vi "ULS ROI.vi"(8 "error in (no error)":errorcluster, 10 "ROI":cluster{"X1":sgl, "X2":sgl, "Y1":sgl, "Y2":sgl}, 11 "IFD in":refnum<class "IFD.lvclass">) -> (0 "error out":errorcluster, 3 "IFD out":refnum<class "IFD.lvclass">)   [LabVIEW 2016, in "IFD.lvclass"]
uses:
  IFD.lvclass
  Tag/IFD_Tag.lvclass/IFD_Tag.ctl
  IFD.lvclass/IFD.ctl
  Tag/IFD_Tag.lvclass
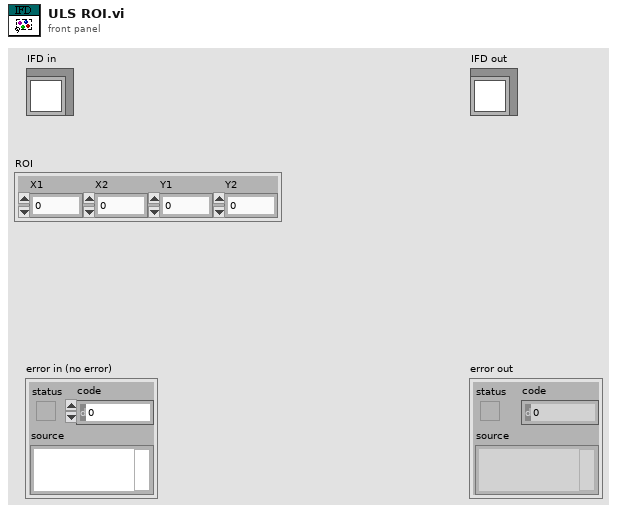
[diagram p1: front panel]
types:
  T1 = enum16{"Undefined(DO NOT USE)", "U8", "ASCII", "U16", "U32", "RATIONAL", "I8", "Undefined 8 bit", "I16", "I32", "SRATIONAL", "SGL", "DBL"}
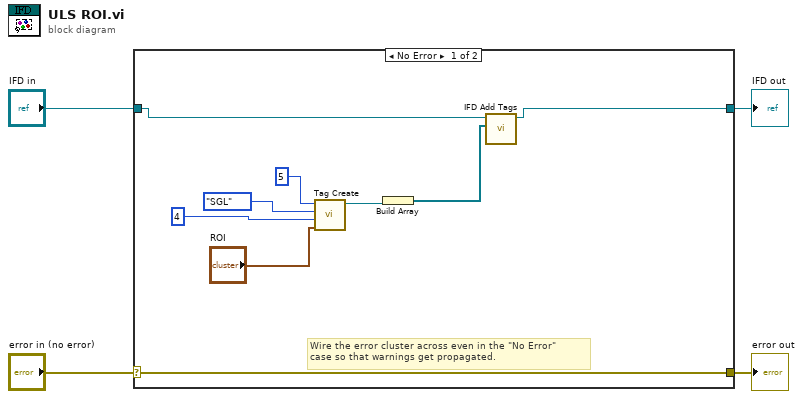
[diagram p0: block diagram]
diagram:
  n1 = case shown="No Error" "error in (no error)" {
    selector: "error in (no error)" -> [w13 w15]
    tunnel: [w13 w15] -> w3
    tunnel: [w10 w14] -> w1
    tunnel: "IFD in" -> [w11 w14]
    frame No Error {
      # "Wire the error cluster across even in the \"No Error\"\ncase so that warnings get propagated."
      n2 = call "Tag Create.vi"("Data"="ROI", "Data Count"=u32 4, "Data Type"=T1."SGL", "Tag ID"=u16 5) -> ("IFD_Tag out"=w12:refnum<class "IFD_Tag.lvclass">)  [unwired: 7 in]
      n3 = Build Array(w12) -> (w9:refnum<class "IFD_Tag.lvclass">[])
      n4 = call "IFD Add Tags.vi"("Tag(s)"=w9, "IFD in"=w11) -> ("IFD out"=w10:refnum<class "IFD.lvclass">)  [unwired: 8 in, 1 out]
    }
    frame Error {
    }
  }
  "error out" <- w3
  "IFD out" <- w1
